vi "Set Viewer Mode.vi"(8 "error in (no error)":errorcluster, 10 "nViewerMode":i32, 11 "lpszDataPath":string) -> (0 "error out":errorcluster, 2 "function return":i32, 3 "lpszDataPath out":string)   [LabVIEW 2017, in "imgAcquisiotn.lvlib"]
doc: "DLLFunction int __stdcall ImageCapSetViewerMode(LPCTSTR lpszDataPath, int nViewerMode);"
uses:
  imgAcquisiotn.lvlib
  lib/ImageCaptureDLL.dll
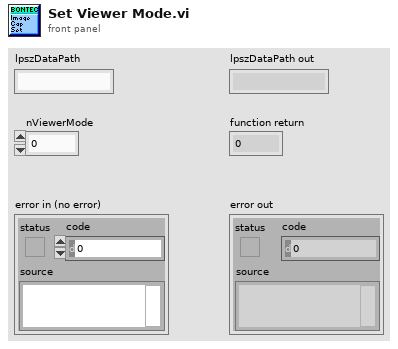
[diagram p1: front panel]
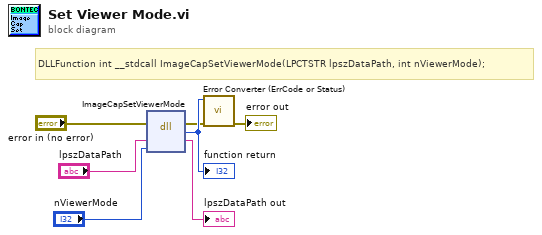
[diagram p0: block diagram]
diagram:
  # "DLLFunction int __stdcall ImageCapSetViewerMode(LPCTSTR lpszDataPath, int nViewerMode);"
  n1 = dll-call lib="F:/BonTechFlatPanelLVDriver/lib/ImageCaptureDLL.*" fn="ImageCapSetViewerMode"(error in="error in (no error)", "lpszDataPath"="lpszDataPath", "nViewerMode"="nViewerMode") -> (error out=w2:errorcluster, w7:i32, "lpszDataPath"=→"lpszDataPath out":string)  [unwired: 3 in, 1 out]
  "function return" <- w7
  n2 = call "Error Converter (ErrCode or Status).vi"("error in (no error)"=w2, "error code"=w7) -> ("error out"=→"error out":errorcluster)  [unwired: 9 in]
